vi "Main Page.vi"(8 "error in (no error)":errorcluster, 11 "Node Ptr":T1 format="%.0x") -> (0 "error out":errorcluster)   [LabVIEW 2017, in "Data Sharing Framework System Explorer.lvlib"]
uses:
  Data Sharing Framework System Explorer.lvlib
  <vilib>/NI Veristand/Custom Device API/Custom Device Item Ref.ctl
  <vilib>/NI Veristand/Custom Device API/Custom Device API.lvlib
  dsf core/Source/DSF Configuration Utility/DSF Configuration Utility.lvlib
panel:
  in  "refresh config":bool
  in  "open_config_viewer":bool
  in  "Path":path
  in  "Header":cluster{"Section Name":string}={"Section Name"="Custom Device Item Settings"}
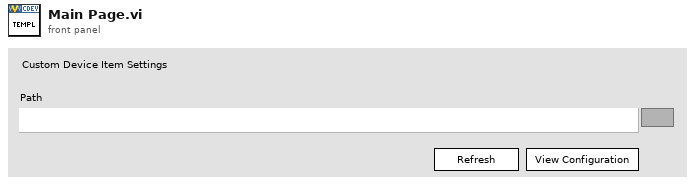
[diagram p1: front panel]
types:
  T1 = typedef "Custom Device API.lvlib/Custom Device Item Ref.ctl" = u64
  T2 = typedef "Custom Device API.lvlib/Custom Device Commands.ctl" = enum16{"Default", "Item renamed", "Shutdown", "Dynamic button pressed"}
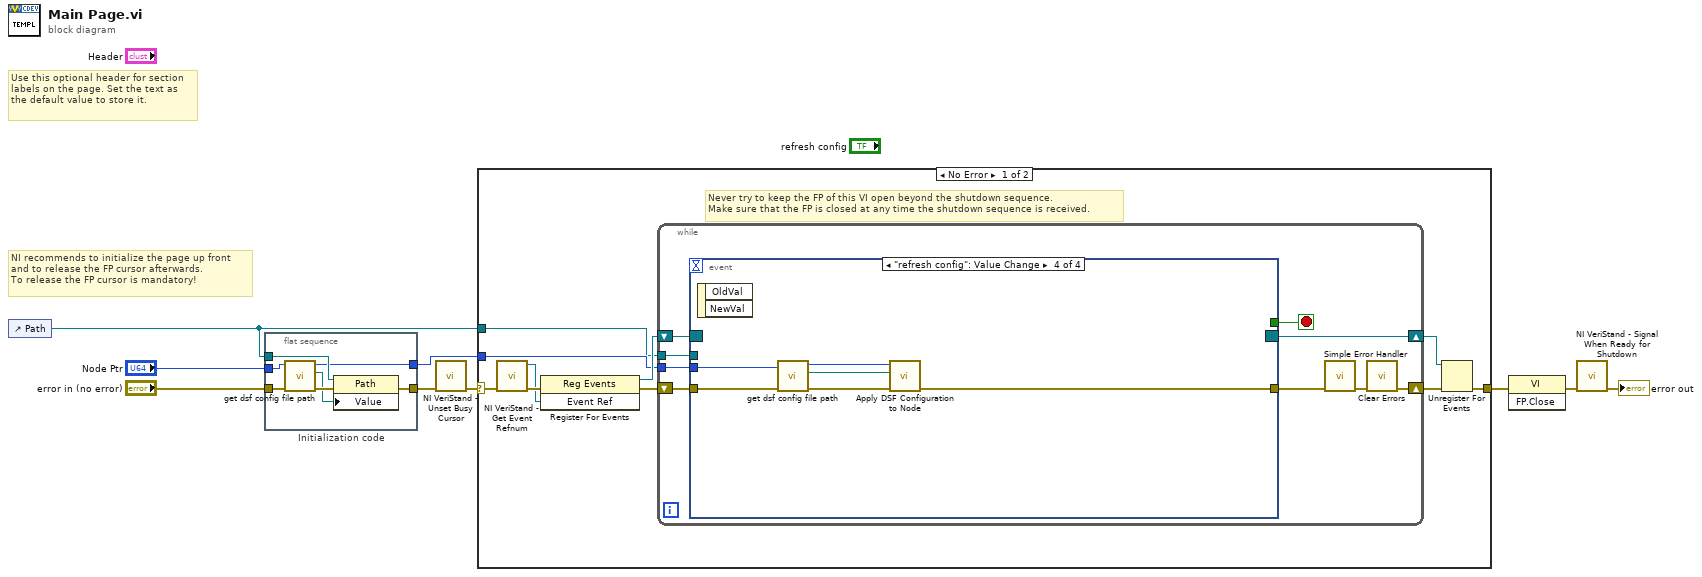
[diagram p0: block diagram]
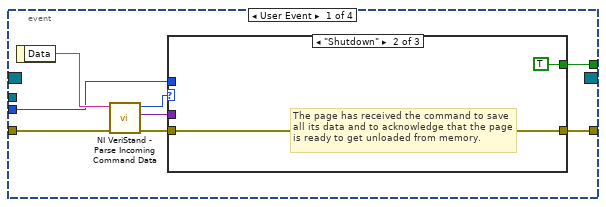
[diagram p2: hidden frame]
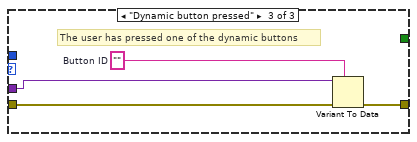
[diagram p4: hidden frame]
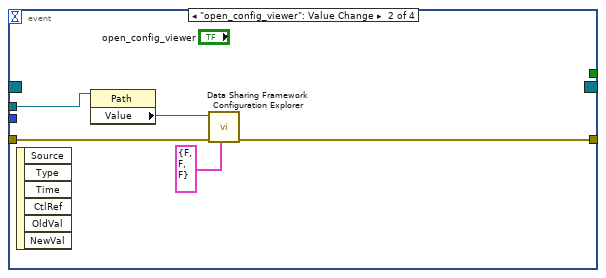
[diagram p5: hidden frame]
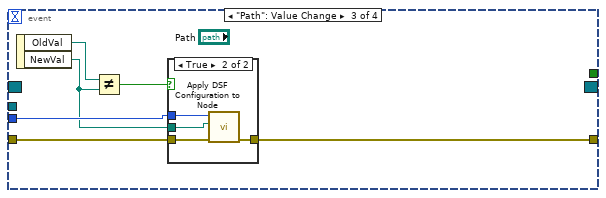
[diagram p6: hidden frame]
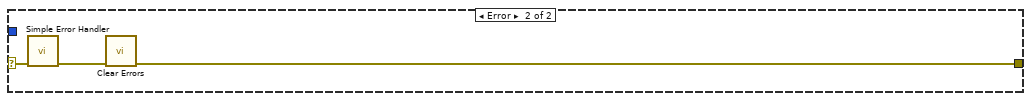
[diagram p8: hidden frame]
diagram:
  # "Use this optional header for section labels on the page. Set the text as the default value to store it."
  # "NI recommends to initialize the page up front\nand to release the FP cursor afterwards.\nTo release the FP cursor is mandatory!"
  n1 = control-ref of="Path"() -> (w1:refnum<vi>)
  n2 = flat-sequence "Initialization code" {
    tunnel: "error in (no error)" -> [w15]
    tunnel: "Node Ptr" -> [w16]
    tunnel: [w13] -> w5
    tunnel: [w11] -> w2
    tunnel: w1 -> [w12]
    frame #0 {
      n3 = call "get dsf config file path.vi"("error in (no error)"=w15, "Node Ptr"=w16) -> ("error out"=w14:errorcluster, "Path"=w10:path, "Item Ref out"=w11:T1)  [unwired: 7 in]
      n4 = property class="Path"(reference=w12, error in=w14, "Value"=w10) -> (error out=w13:errorcluster)  [unwired: 1 out]
    }
  }
  n5 = call <vilib>:"NI VeriStand - Unset Busy Cursor.vi"("error in (no error)"=w5) -> ("error out"=w4:errorcluster)  [unwired: 10 out]
  n6 = case shown="No Error" w4 {
    selector: w4 -> [w18 w75]
    tunnel: [w23 w73] -> w9
    tunnel: w2 -> [w19 _]
    tunnel: w1 -> [w17 _]
    frame No Error {
      # "Never try to keep the FP of this VI open beyond the shutdown sequence.\nMake sure that the FP is closed at any time the shutdown sequence is received."
      n7 = call <vilib>:"NI VeriStand - Get Event Refnum.vi"("error in (no error)"=w18) -> ("error out"=w26:errorcluster, "Event Ref"=w22:refnum<user-event>)  [unwired: 9 out]
      n8 = register-events(error in=w26, w22) -> (reference out=w20:refnum<event-registration>, error out=w21:errorcluster)  [unwired: 1 in]
      n9 = while {
        tunnel: w19 -> [w31]
        shift-right: [w28] -> w24
        shift-left: w21 -> [w34]
        shift-right: [w35] -> w25
        shift-left: w20 -> [w33]
        tunnel: w17 -> [w27]
        stop <- w32 stop-if-true
        n10 = event shown="[3] \"refresh config\": Value Change" {
          selector: w33 -> [_ _ _ _]
          dyn-events: [_ _ _ _] -> w35
          timeout: _ -> [_ _ _ _]
          tunnel: w34 -> [w43 w55 w61 w72]
          tunnel: [w39 _ _ _] -> w32
          tunnel: [w38 w54 w59 w71] -> w30
          tunnel: w31 -> [w37 _ w60 w69]
          tunnel: w27 -> [_ w53 _ _]
          event User Event {
            n11 = event-data() -> ("Data"=w42:string)  [unwired: 1 out]
            n12 = call <vilib>:"NI VeriStand - Parse Incoming Command Data.vi"("error in (no error)"=w43, "Incoming data"=w42) -> ("error out"=w41:errorcluster, "Outgoing data"=w36:variant, "Action"=w40:T2)  [unwired: 7 out]
            n13 = case shown="\"Shutdown\"" w40 {
              tunnel: w41 -> [w44 w45 w50]
              tunnel: [_ TRUE _] -> w39
              tunnel: [w44 w45 w47] -> w38
              tunnel: w37 -> [_ _ _]
              tunnel: w36 -> [_ _ w49]
              frame "Default", Default {
              }
              frame "Shutdown" {
                # "The page has received the command to save all its data and to acknowledge that the page is ready to get unloaded from memory."
              }
              frame "Dynamic button pressed" {
                w48 = ""  # Button ID
                # "The user has pressed one of the dynamic buttons"
                n14 = Variant To Data(error in=w50, type=w48, Variant=w49) -> (error out=w47:errorcluster)  [unwired: 1 out]
              }
            }
          }
          event "open_config_viewer": Value Change {
            n15 = event-data() -> ()  [unwired: 7 out]
            n16 = property class="Path"(reference=w53) -> ("Value"=w52:path)  [unwired: 1 in, 2 out]
            n17 = call "Data Sharing Framework Configuration Explorer.vi"("menu options"=cluster{"open":bool, "save":bool, "view":bool} {"open"=FALSE, "save"=FALSE, "view"=FALSE}, "error in (no error)"=w55, "Path in"=w52) -> ("error out"=w54:errorcluster)  [unwired: 7 in, 1 out]
          }
          event "Path": Value Change {
            n18 = event-data() -> ("OldVal"=w58:path, "NewVal"=w57:path)  [unwired: 1 out]
            n19 = Not Equal?(x=w58, y=w57) -> (x != y?=w56:bool)
            n20 = case shown="True" w56 {
              tunnel: w61 -> [w62 w66]
              tunnel: w60 -> [_ w63]
              tunnel: [w62 w65] -> w59
              tunnel: w57 -> [_ w64]
              frame False {
              }
              frame True {
                n21 = call "Apply DSF Configuration to Node.vi"("error in (no error)"=w66, "NewVal"=w64, "Item Ref in"=w63) -> ("error out"=w65:errorcluster)  [unwired: 8 in]
              }
            }
          }
          event "refresh config": Value Change {
            n22 = event-data() -> ()  [unwired: 3 out]
            n23 = call "get dsf config file path.vi"("error in (no error)"=w72, "Node Ptr"=w69) -> ("error out"=w70:errorcluster, "Path"=w67:path, "Item Ref out"=w68:T1)  [unwired: 7 in]
            n24 = call "Apply DSF Configuration to Node.vi"("error in (no error)"=w70, "NewVal"=w67, "Item Ref in"=w68) -> ("error out"=w71:errorcluster)  [unwired: 8 in]
          }
        }
        n25 = call <vilib>:"Simple Error Handler.vi"("error in (no error)"=w30) -> ("error out"=w29:errorcluster)  [unwired: 1 in, 7 out]
        n26 = call <vilib>:"Clear Errors.vi"("error in (no error)"=w29) -> ("error out"=w28:errorcluster)  [unwired: 1 in, 5 out]
      }
      n27 = Unregister For Events(event registration refnum=w25, error in=w24) -> (error out=w23:errorcluster)
    }
    frame Error {
      n28 = call <vilib>:"Simple Error Handler.vi"("error in (no error)"=w75) -> ("error out"=w74:errorcluster)  [unwired: 1 in, 7 out]
      n29 = call <vilib>:"Clear Errors.vi"("error in (no error)"=w74) -> ("error out"=w73:errorcluster)  [unwired: 1 in, 5 out]
    }
  }
  n30 = invoke class="VI" method="FP.Close"(error in=w9) -> (error out=w8:errorcluster)  [unwired: 2 in, 2 out]
  n31 = call <vilib>:"NI VeriStand - Signal When Ready for Shutdown.vi"("error in (no error)"=w8) -> ("error out"=→"error out":errorcluster)  [unwired: 10 out]
